vi "Clear Config Tree.vi"(8 "error in":errorcluster, 9 "Chassis Name":string, 10 "ChassisType":T1, 11 "FP Controls in":refnum<class "FP Controls.lvclass">) -> (0 "error out":errorcluster, 3 "FP Controls out":refnum<class "FP Controls.lvclass">)   [LabVIEW 2018, in "Configuration Grandmaster.lvlib" / "FP Controls.lvclass"]
uses:
  FP Controls.lvclass
  Common/Controls/Chassis Type.ctl
  FP Controls.lvclass/FP Controls.ctl
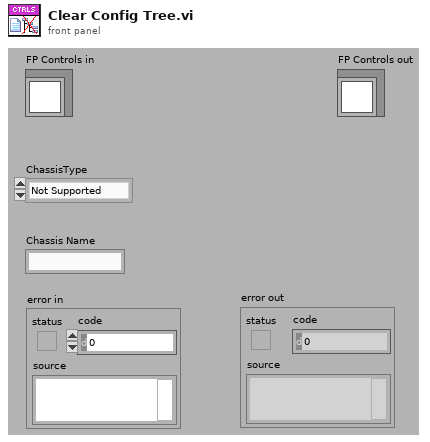
[diagram p1: front panel]
types:
  T1 = typedef "Chassis Type.ctl" = enum16{"Not Supported", "C Series 1-Slot", "C Series 4-Slot", "C Series 8-Slot", "PXI 8-Slot", "PXIe 18-Slot"}
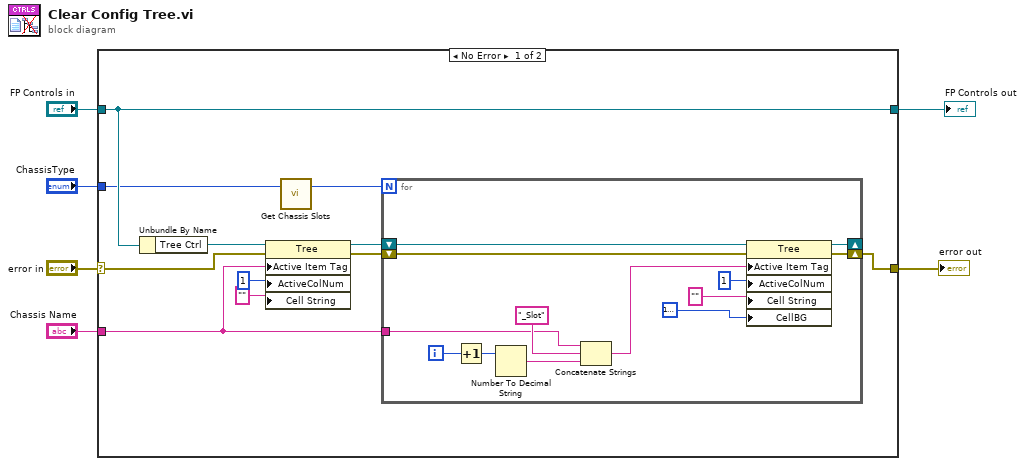
[diagram p0: block diagram]
diagram:
  n1 = case shown="No Error" "error in" {
    selector: "error in" -> [w9 w31]
    tunnel: "ChassisType" -> [w8 _]
    tunnel: "Chassis Name" -> [w13 _]
    tunnel: [w12 w31] -> w4
    tunnel: "FP Controls in" -> [w10 w32]
    tunnel: [w10 w32] -> w2
    frame No Error {
      n2 = Unbundle By Name(w10) -> ("Tree Ctrl"=w11:refnum<vi>)
      n3 = property class="Tree"(reference=w11, error in=w9, "Active Item Tag"=w13, "ActiveColNum"=1 ("Active Cell:Active Column Number"), "Cell String"="" ("Active Cell:String")) -> (reference out=w15:refnum<vi>, error out=w16:errorcluster)
      n4 = call "Get Chassis Slots.vi"("ChassisType"=w8) -> ("Num of Slots"=w7:i32)  [unwired: 2 in]
      n5 = for {
        N: w7 -> [_]
        shift-right: [w29] -> w12
        shift-left: w16 -> [w20]
        shift-right: [w30] -> _
        shift-left: w15 -> [w21]
        tunnel: w13 -> [w25]
        i -> [w23]
        n6 = Increment(x=w23) -> (x+1=w24:i32)
        n7 = Number To Decimal String(number=w24) -> (decimal integer string=w28:string)  [unwired: 1 in]
        n8 = Concatenate Strings(w25, "_Slot" ("string"), w28) -> (w22:string)
        n9 = property class="Tree"(reference=w21, error in=w20, "Active Item Tag"=w22, "ActiveColNum"=1 ("Active Cell:Active Column Number"), "Cell String"="" ("Active Cell:String"), "CellBG"=u32 16777225) -> (reference out=w30:refnum<vi>, error out=w29:errorcluster)
      }
    }
    frame Error {
    }
  }
  "error out" <- w4
  "FP Controls out" <- w2
